vi "Create.vi"(8 "error in (no error)":errorcluster, 10 "messageID":u16) -> (0 "error out":errorcluster, 3 "mqttCmdPublishComplete out":refnum<class "PublishCompleteMqttMsg.lvclass">)   [LabVIEW 2020, in "PublishCompleteMqttMsg.lvclass"]
uses:
  PublishCompleteMqttMsg.lvclass
  PublishCompleteMqttMsg.lvclass/PublishCompleteMqttMsg.ctl
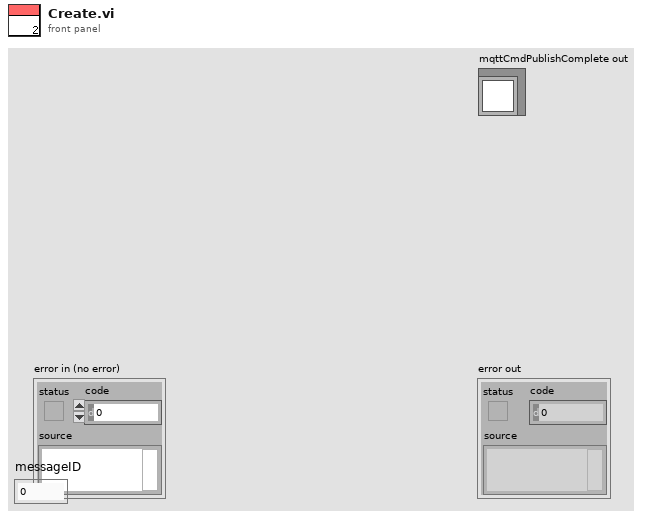
[diagram p1: front panel]
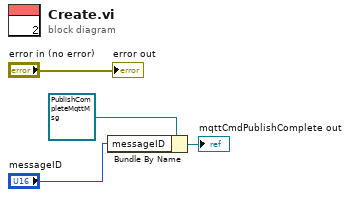
[diagram p0: block diagram]
diagram:
  n1 = Bundle By Name(cluster=refnum<class "PublishCompleteMqttMsg.lvclass"> refnum ("mqttCmdPublishComplete in"), "messageID"="messageID") -> (→"mqttCmdPublishComplete out":refnum<class "PublishCompleteMqttMsg.lvclass">)
  "error out" <- "error in (no error)"
